vi "Read Sub Panel Message.vi"(8 "error in (no error)":errorcluster, 11 "MSG in":refnum<class "MSG.lvclass">) -> (0 "error out":errorcluster, 2 "Sub Panel Message":refnum<vi>, 3 "MSG out":refnum<class "MSG.lvclass">)   [LabVIEW 2020, in "MSG.lvlib" / "MSG.lvclass"]
uses:
  MSG.lvclass
  MSG.lvclass/MSG.ctl
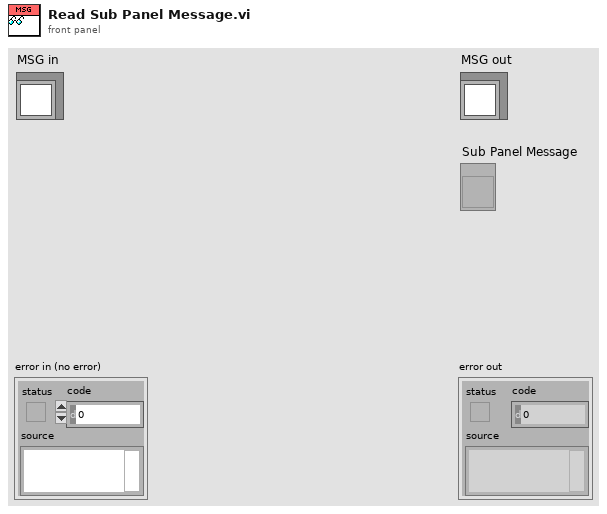
[diagram p1: front panel]
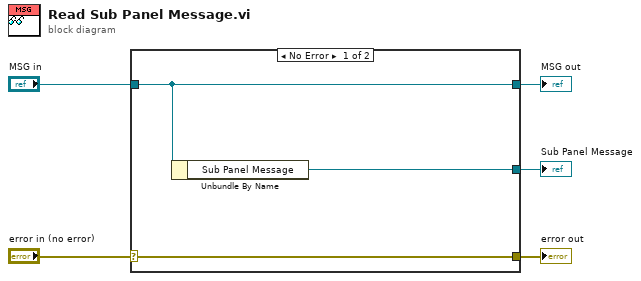
[diagram p0: block diagram]
diagram:
  n1 = case shown="No Error" "error in (no error)" {
    selector: "error in (no error)" -> [w8 w9]
    tunnel: [w8 w9] -> w4
    tunnel: [w7 w10] -> w2
    tunnel: "MSG in" -> [w7 w10]
    tunnel: [w6 _] -> w1
    frame No Error {
      n2 = Unbundle By Name(w7) -> ("Sub Panel Message"=w6:refnum<vi>)
    }
    frame Error {
    }
  }
  "error out" <- w4
  "MSG out" <- w2
  "Sub Panel Message" <- w1
